vi "Encoder Read.vi"() -> (0 "Encoder Position":dbl format="%.3f")   [LabVIEW 2009]
uses:
  TMC Global.vi
panel:
  out "Iterations":i32
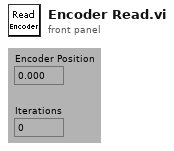
[diagram p1: front panel]
types:
  T1 = cluster{"input XON/XOFF":bool, "input HW Handshake":bool, "input alt HW HShk":bool, "output XON/XOFF":bool, "output HW Handshake":bool, "output alt HW HShk":bool, "XOFF byte":u8, "XON byte":u8, "parity error byte":u16}
  T2 = enum16{"no parity", "odd parity", "even parity", "mark parity", "space parity"}
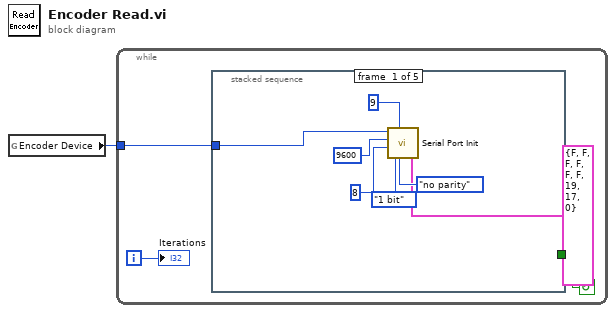
[diagram p0: block diagram]
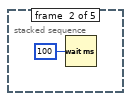
[diagram p2: hidden frame]
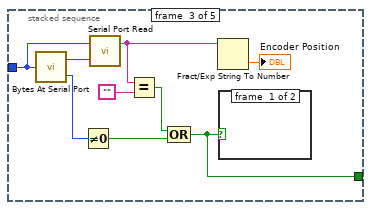
[diagram p3: hidden frame]
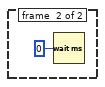
[diagram p4: hidden frame]
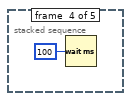
[diagram p5: hidden frame]
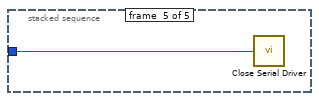
[diagram p6: hidden frame]
diagram:
  n1 = global read "TMC Global.vi" "Encoder Device"() -> (w1:i32)
  n2 = while {
    tunnel: w1 -> [w4]
    i -> [w2]
    stop <- w3 continue-if-true
    n3 = stacked-sequence {
      tunnel: w4 -> [w5 _ w21 _ w24]
      tunnel: [_ _ w13 _ _] -> w3
      frame #0 {
        n4 = call <vilib>:"Serial Port Init.vi"("flow control etc."=T1 {"input XON/XOFF"=FALSE, "input HW Handshake"=FALSE, "input alt HW HShk"=FALSE, "output XON/XOFF"=FALSE, "output HW Handshake"=FALSE, "output alt HW HShk"=FALSE, "XOFF byte"=19, "XON byte"=17, "parity error byte"=0}, "parity"=T2."no parity", "buffer size"=u16 9, "stop bits"=enum16{"1 bit", "1.5 bits", "2 bits"}."1 bit", "data bits"=u16 8, "baud rate"=u32 9600, "port number"=w5) -> ()  [unwired: 1 out]
      }
      frame #1 {
        n5 = Wait (ms)(milliseconds to wait=u32 100) -> ()  [unwired: 1 out]
      }
      frame #2 {
        n6 = call <vilib>:"Bytes At Serial Port.vi"("port number"=w21) -> ("byte count"=w14:u32, "error code"=w17:i32)
        n7 = Not Equal To 0?(x=w17) -> (x != 0?=w18:bool)
        n8 = call <vilib>:"Serial Port Read.vi"("requested byte count"=w14, "port number"=w21) -> ("string read"=w19:string)  [unwired: 1 out]
        n9 = Equal?(x=w19, y="") -> (x = y?=w15:bool)
        n10 = Compound Arithmetic op=OR(w15, w18) -> (w13:bool)
        n11 = Fract/Exp String To Number(string=w19) -> (number=→"Encoder Position":dbl)  [unwired: 3 in, 1 out]
        n12 = case shown="True" w13 {
          frame #0 {
          }
          frame #1 {
            n13 = Wait (ms)(milliseconds to wait=u32 0) -> ()  [unwired: 1 out]
          }
        }
      }
      frame #3 {
        n14 = Wait (ms)(milliseconds to wait=u32 100) -> ()  [unwired: 1 out]
      }
      frame #4 {
        n15 = call <vilib>:"Close Serial Driver.vi"("port number"=w24) -> ()  [unwired: 1 out]
      }
    }
    "Iterations" <- w2
  }
